vi "Real Hb Filter - 8 spc.vi"(0 "input data":fxp<+/-,18,1>[](array[numeric])=[-0.00127410888671875, 0.0, 0.0, 0.0, 0.0, 0.0, 0.0, 0.0], 7 "coefficients":fxp<+/-,18,1>[](array[numeric])=[-0.00127410888671875, 0.00325775146484375, -0.0070953369140625, 0.01354217529296875, -0.02376556396484375, 0.03955841064453125, -0.0644073486328125, 0.10701751708984375, -0.1994476318359375, 0.6322708129882812]) -> (4 "output data":fxp<+/-,18,1>[](array[numeric]))   [LabVIEW 2019]
uses:
  <vilib>/rvi/FXPMathLib/basic elements/FxpDiscreteDelay/XNode/nifxpmath_DiscreteDelay.xnode
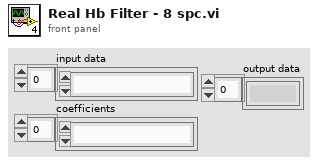
[diagram p1: front panel]
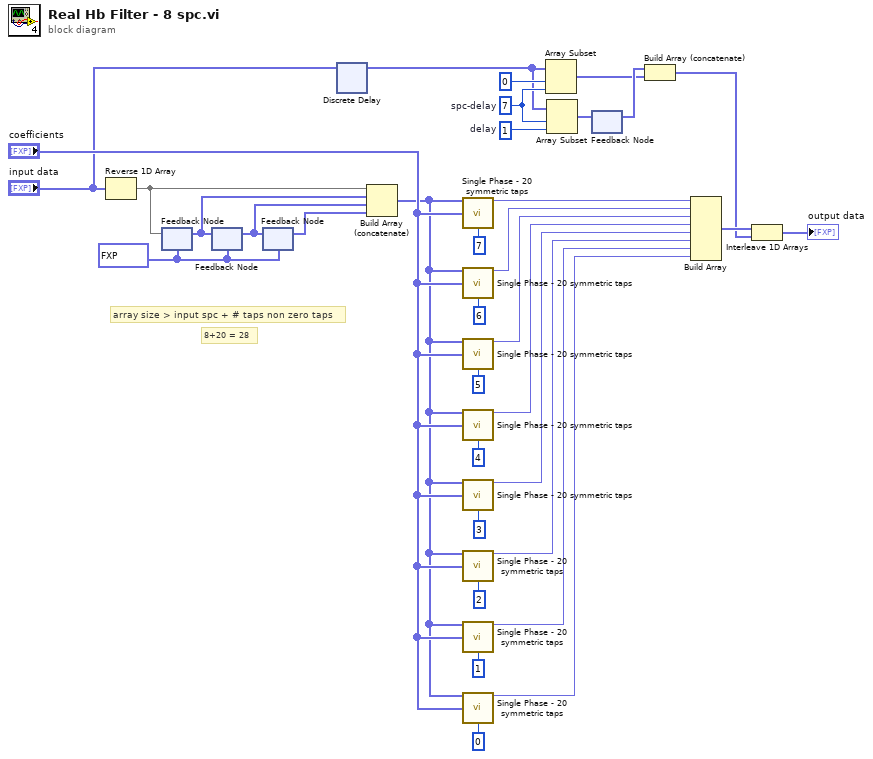
[diagram p0: block diagram]
diagram:
  w3 = 7  # spc-delay
  w4 = 1  # delay
  w10 = fxp<+/-,18,1>[] [0.0, 0.0, 0.0, 0.0, 0.0, 0.0, 0.0, 0.0]
  # "8+20 = 28"
  # "array size > input spc + # taps non zero taps"
  n1 = Reverse 1D Array(array="input data") -> (reversed array=w14:fxp<+/-,18,1>[])
  n2 = feedback-in #1(w14) -> ()
  n3 = feedback #1(w10) -> (w34:fxp<+/-,18,1>[])
  n4 = feedback #2(w10) -> (w33:fxp<+/-,18,1>[])
  n5 = feedback-in #2(w34) -> ()
  n6 = feedback #3(w10) -> (w32:fxp<+/-,18,1>[])
  n7 = feedback-in #3(w33) -> ()
  n8 = xnode "Discrete Delay"("D"="input data") -> ("Q"=w1:fxp<+/-,18,1>[])
  n9 = Build Array (concatenate)(w14, w34, w33, w32) -> (w13:fxp<+/-,18,1>[])
  n10 = call "Single Phase - 20 symmetric taps.vi"("input data"=w13, "coefficients"="coefficients", "phase"=i16 7) -> ("output data"=w22:fxp<+/-,18,1>)  [unwired: 12 in]
  n11 = call "Single Phase - 20 symmetric taps.vi"("input data"=w13, "coefficients"="coefficients", "phase"=i16 6) -> ("output data"=w21:fxp<+/-,18,1>)  [unwired: 12 in]
  n12 = call "Single Phase - 20 symmetric taps.vi"("input data"=w13, "coefficients"="coefficients", "phase"=i16 5) -> ("output data"=w20:fxp<+/-,18,1>)  [unwired: 12 in]
  n13 = call "Single Phase - 20 symmetric taps.vi"("input data"=w13, "coefficients"="coefficients", "phase"=i16 4) -> ("output data"=w19:fxp<+/-,18,1>)  [unwired: 12 in]
  n14 = call "Single Phase - 20 symmetric taps.vi"("input data"=w13, "coefficients"="coefficients", "phase"=i16 3) -> ("output data"=w18:fxp<+/-,18,1>)  [unwired: 12 in]
  n15 = call "Single Phase - 20 symmetric taps.vi"("input data"=w13, "coefficients"="coefficients", "phase"=i16 2) -> ("output data"=w17:fxp<+/-,18,1>)  [unwired: 12 in]
  n16 = call "Single Phase - 20 symmetric taps.vi"("input data"=w13, "coefficients"="coefficients", "phase"=i16 1) -> ("output data"=w16:fxp<+/-,18,1>)  [unwired: 12 in]
  n17 = call "Single Phase - 20 symmetric taps.vi"("input data"=w13, "coefficients"="coefficients", "phase"=i16 0) -> ("output data"=w15:fxp<+/-,18,1>)  [unwired: 12 in]
  n18 = Array Subset(array=w1, index=0, length=w3) -> (w7:fxp<+/-,18,1>[])
  n19 = Array Subset(array=w1, index=w3, length=w4) -> (w9:fxp<+/-,18,1>[])
  n20 = feedback #4() -> (w8:fxp<+/-,18,1>[])  [unwired: 1 in]
  n21 = feedback-in #4(w9) -> ()
  n22 = Build Array (concatenate)(w8, w7) -> (w5:fxp<+/-,18,1>[])
  n23 = Build Array(w22, w21, w20, w19, w18, w17, w16, w15) -> (w12:fxp<+/-,18,1>[])
  n24 = Interleave 1D Arrays(w12, w5) -> (→"output data":fxp<+/-,18,1>[])
